vi "Compile Knock Cylinder 1.0 Data.vi"(7 "RIO Address":string, 8 "error in (no error)":errorcluster, 11 "Device Item Ref in":T3 format="%.0x") -> (0 "error out":errorcluster, 2 "Knock Cylinders":T1[](array[typedef]), 3 "Device Item Ref out":T3 format="%.0x")   [LabVIEW 2020, in "Engine Simulation Toolkit System Explorer.lvlib"]
uses:
  Engine Simulation Toolkit System Explorer.lvlib
  <vilib>/NI VeriStand/Custom Device API/Custom Device Item Ref.ctl
  Shared/1.0 Knock Cylinder Engine Data.ctl
  Shared/1.0 Knock Cylinder FIFO Idxs.ctl
  Shared/Constants and GUIDs.vi
  <vilib>/NI VeriStand/Custom Device Tools/Custom Device Utility Library/NI VeriStand - Search for Item by GUID.vi
  Shared/Properties.vi
  <vilib>/NI VeriStand/Custom Device API/Get Item Property (Double).vi
  <vilib>/NI VeriStand/Custom Device API/Get Item Property (String).vi
  Shared/Engine Simulation Toolkit Shared.lvlib
  <vilib>/NI VeriStand/Custom Device Tools/Custom Device Utility Library/Custom Device Utility Library.lvlib
  <vilib>/NI VeriStand/Custom Device API/Custom Device API.lvlib
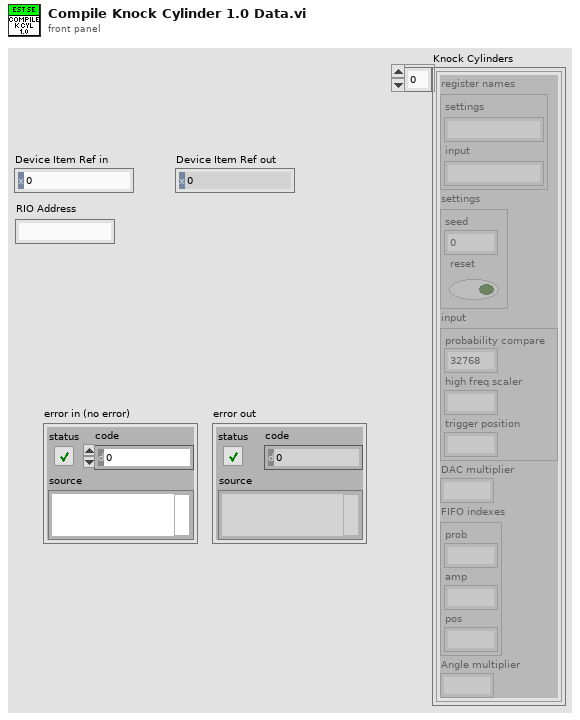
[diagram p1: front panel]
types:
  T1 = typedef "Engine Simulation Toolkit Shared.lvlib/1.0 Knock Cylinder Engine Data.ctl" = cluster{"register names":cluster{"settings":string, "input":string}, "settings":cluster{"seed":u16, "reset":bool}, "input":cluster{"probability compare":u16, "high freq scaler":fxp<+,10,0>, "trigger position":u16}, "DAC multiplier":dbl, "FIFO indexes":T2, "Angle multiplier":dbl}
  T2 = typedef "Engine Simulation Toolkit Shared.lvlib/1.0 Knock Cylinder FIFO Idxs.ctl" = cluster{"prob":i32, "amp":i32, "pos":i32}
  T3 = typedef "Custom Device API.lvlib/Custom Device Item Ref.ctl" = u64
  T4 = typedef "Engine Simulation Toolkit Shared.lvlib/Channel.ctl" = cluster{"Name":string, "Units":string, "Default":dbl, "Description":string, "Scalable":bool}
  T5 = typedef "Engine Simulation Toolkit System Explorer.lvlib/Knock Cylinder.ctl" = cluster{"Name":string, "Bitfile name":string, "Probability":dbl, "Amplitude":dbl, "Angle":dbl}
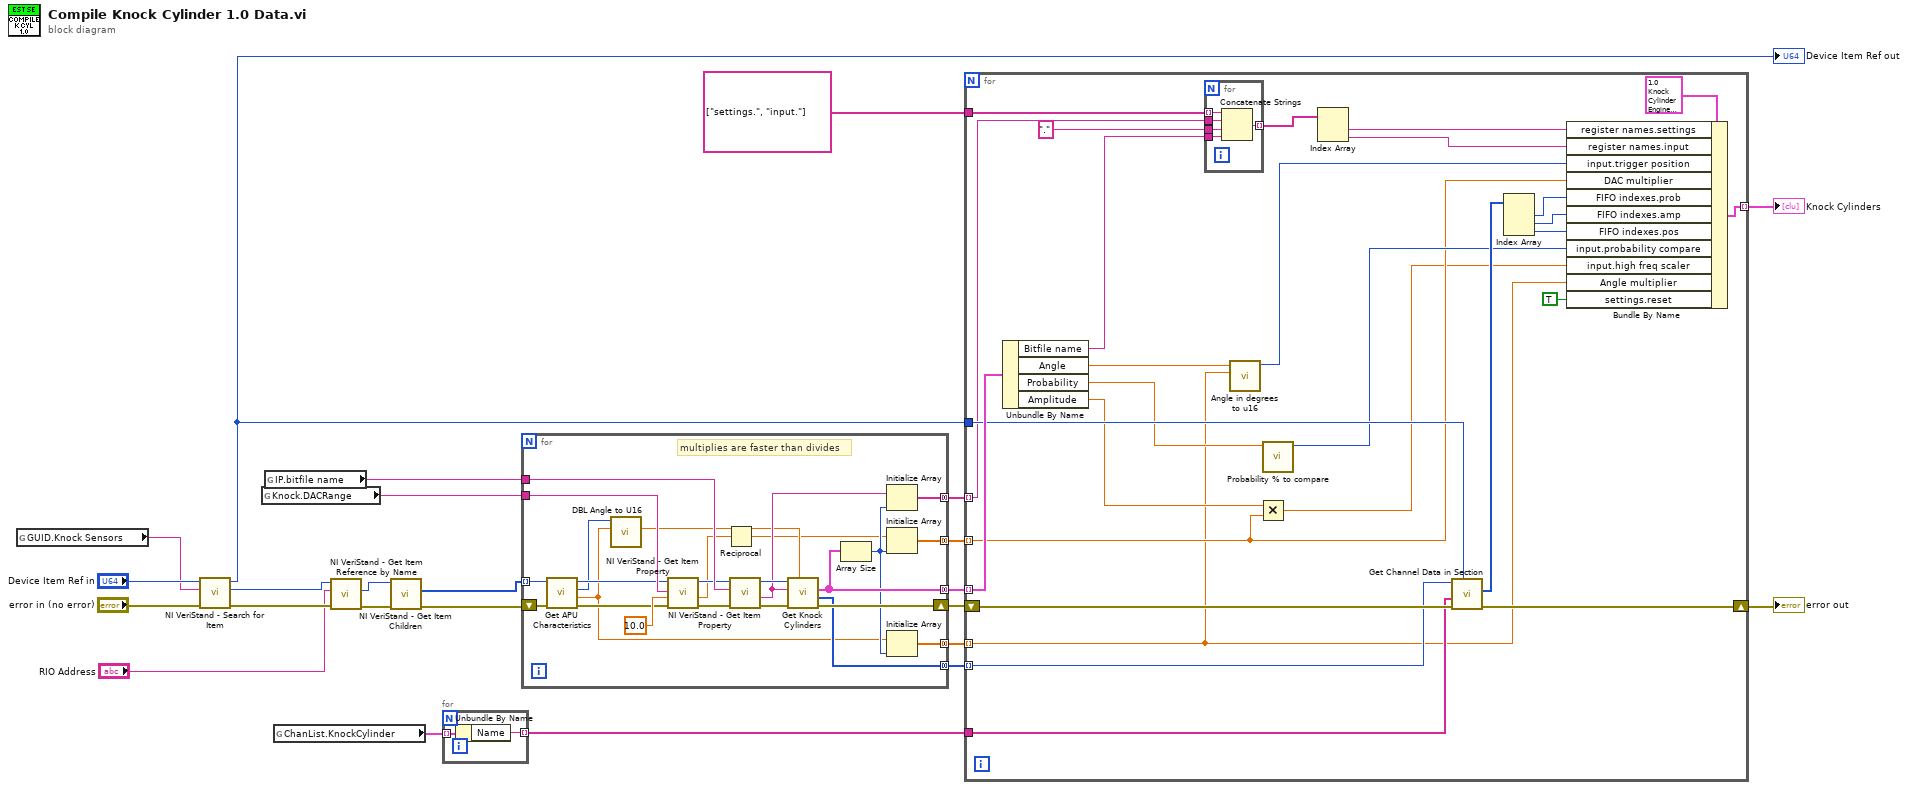
[diagram p0: block diagram]
diagram:
  n1 = global read "Constants and GUIDs.vi" "GUID.Knock Sensors"() -> (w16:string)
  n2 = call-poly <vilib>:"NI VeriStand - Search for Item.vi"("error in"="error in (no error)", "Item GUID"=w16, "Section Ref in"="Device Item Ref in") -> ("error out"=w4:errorcluster, "Item Ref"=w5:T3, "Section Ref out"=w19:T3)  [unwired: 5 in, 1 out]
  "Device Item Ref out" <- w19
  n3 = global read "Properties.vi" "Knock.DACRange"() -> (w14:string)
  n4 = global read "Properties.vi" "IP.bitfile name"() -> (w13:string)
  n5 = global read "Constants and GUIDs.vi" "ChanList.KnockCylinder"() -> (w18:T4[])
  n6 = call <vilib>:"NI VeriStand - Get Item Reference by Name.vi"("error in (no error)"=w4, "Item Name"="RIO Address", "Parent Ref in"=w5) -> ("error out"=w6:errorcluster, "Item Ref"=w7:T3)  [unwired: 5 in, 2 out]
  n7 = call <vilib>:"NI VeriStand - Get Item Children.vi"("error in (no error)"=w6, "Item Ref in"=w7) -> ("error out"=w3:errorcluster, "Child Refs"=w2:T3[])  [unwired: 6 in, 2 out]
  n8 = for {
    tunnel: w18 -> [w26] mode=indexing
    tunnel: [w25] -> w17 mode=indexing
    n9 = Unbundle By Name(w26) -> ("Name"=w25:string)
  }
  n10 = for {
    tunnel: w2 -> [w34] mode=indexing
    shift-right: [w45] -> w15
    shift-left: w3 -> [w50]
    tunnel: w14 -> [w47]
    tunnel: w13 -> [w46]
    tunnel: [w43] -> w12 mode=concatenating
    tunnel: [w38] -> w11 mode=concatenating
    tunnel: [w42] -> w10 mode=concatenating
    tunnel: [w41] -> w9 mode=concatenating
    tunnel: [w28] -> w8 mode=concatenating
    # "multiplies are faster than divides"
    n11 = call "Get APU Characteristics.vi"("error in (no error)"=w50, "Item Ref in"=w34) -> ("error out"=w35:errorcluster, "angle to u16 scale factor"=w29:dbl, "total angle span (degrees)"=w32:u16, "Item Ref out"=w33:T3)  [unwired: 3 in, 3 out]
    n12 = call "DBL Angle to U16.vi"("angle to u16 scale factor"=w29, "Desired angle (degrees)"=w32) -> ("Actual angle (degrees)"=w31:dbl)  [unwired: 8 in, 1 out]
    n13 = call-poly <vilib>:"NI VeriStand - Get Item Property.vi"("error in (no error)"=w35, "Default Value"=10.0, "Property Name"=w47, "Item Ref in"=w33) -> ("error out"=w49:errorcluster, "Value"=w36:dbl, "Item Ref out"=w40:T3)  [unwired: 4 in, 1 out]
    n14 = Reciprocal(x=w36) -> (1/x=w27:dbl)
    n15 = call-poly <vilib>:"NI VeriStand - Get Item Property.vi"("error in (no error)"=w49, "Property Name"=w46, "Item Ref in"=w40) -> ("error out"=w48:errorcluster, "Value"=w39:string, "Item Ref out"=w44:T3)  [unwired: 5 in, 1 out]
    n16 = call "Get Knock Cylinders.vi"("Max angle"=w31, "error in (no error)"=w48, "Knock Sensor"=w39, "Item Ref in"=w44) -> ("error out"=w45:errorcluster, "cylinder item refs"=w38:T3[], "cylinders"=w43:T5[])  [unwired: 3 in, 2 out]
    n17 = Array Size(array=w43) -> (size(s)=w30:i32)
    n18 = Initialize Array(w39, w30) -> (w41:string[])
    n19 = Initialize Array(w27, w30) -> (w42:dbl[])
    n20 = Initialize Array(w29, w30) -> (w28:dbl[])
  }
  n21 = for {
    shift-right: [w67] -> w21
    shift-left: w15 -> [w71]
    tunnel: string[] ["settings.", "input."] -> [w78]
    tunnel: w17 -> [w68]
    tunnel: [w76] -> w20 mode=indexing
    tunnel: w19 -> [w69]
    tunnel: w12 -> [w75] mode=indexing
    tunnel: w11 -> [w70] mode=indexing
    tunnel: w10 -> [w55] mode=indexing
    tunnel: w9 -> [w64] mode=indexing
    tunnel: w8 -> [w52] mode=indexing
    n22 = Unbundle By Name(w75) -> ("Bitfile name"=w74:string, "Angle"=w62:dbl, "Probability"=w58:dbl, "Amplitude"=w56:dbl)
    n23 = for {
      tunnel: w78 -> [w83] mode=indexing
      tunnel: [w79] -> w73 mode=indexing
      tunnel: w74 -> [w82]
      tunnel: w64 -> [w81]
      tunnel: "." -> [w80]
      n24 = Concatenate Strings(w83, w81, w80, w82) -> (w79:string)
    }
    n25 = call "Angle in degrees to u16.vi"("angle to u16 scale factor"=w52, "Angle (deg)"=w62) -> ("u16 angle"=w61:u16)  [unwired: 8 in, 1 out]
    n26 = Multiply(x=w56, y=w55) -> (x*y=w54:dbl)
    n27 = call "Probability % to compare.vi"("probability %"=w58) -> ("probability compare"=w57:u16)  [unwired: 10 in]
    n28 = Index Array(array=w73) -> (element #1=w72:string, element #2=w63:string)  [unwired: 2 in]
    n29 = call "Get Channel Data in Section.vi"("Custom device ref"=w69, "error in (no error)"=w71, "Channels"=w68, "Item Ref in"=w70) -> ("error out"=w67:errorcluster, "FIFO indexes"=w66:i32[])  [unwired: 3 in, 3 out]
    n30 = Index Array(array=w66) -> (element #1=w60:i32, element #2=w59:i32, element #3=w53:i32)  [unwired: 3 in]
    n31 = Bundle By Name(cluster=T1 {"register names"={"settings"="", "input"=""}, "settings"={"seed"=0, "reset"=FALSE}, "input"={"probability compare"=32768, "high freq scaler"=0.0, "trigger position"=0}, "DAC multiplier"=0.0, "FIFO indexes"={"prob"=0, "amp"=0, "pos"=0}, "Angle multiplier"=0.0} ("1.0.0 Knock Cylinder"), "register names.settings"=w72, "register names.input"=w63, "input.trigger position"=w61, "DAC multiplier"=w55, "FIFO indexes.prob"=w60, "FIFO indexes.amp"=w59, "FIFO indexes.pos"=w53, "input.probability compare"=w57, "input.high freq scaler"=w54, "Angle multiplier"=w52, "settings.reset"=TRUE) -> (w76:T1)
  }
  "error out" <- w21
  "Knock Cylinders" <- w20
